vi "FRC myRIO v1.0 Write I2C.vi"(4 "Keep Bus Busy":bool, 6 "Slave Address (7-bit)":u8, 7 "Timeout ms (5)":i32=5, 8 "Error In (No Error)":errorcluster, 9 "Data to Write":u8[](array[numeric])) -> (0 "error out":errorcluster)   [LabVIEW 2017]
uses:
  <vilib>/rvi/errors/niLvFpgaAdjustHostInterfaceError.vi
  <vilib>/Rock Robotics/SystemInterfaces/System/FPGA_SystemFRC FPGA Ref.ctl
  <vilib>/rvi/interface/nirviReadWriteControl/nirviReadWriteControl.xnode
  NiFpgaLv.dll
  <vilib>/rvi/interface/Simulation/niFpgaSimulationCallBeginRW.vi
panel:
  # "This VI writes an array of data to the SPI Data Out register (SPIn.SPDO) and reads an array of data from the SPI Data In register (SPIn.SPDI) for a particular SPI channel (n). The data is written/read one value at a time. Please see Block Diagram for details."
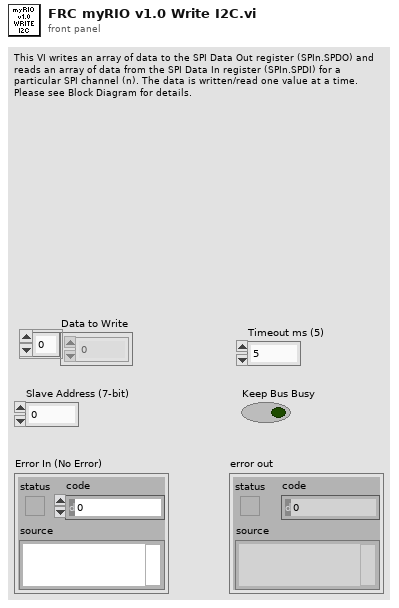
[diagram p1: front panel]
types:
  T1 = typedef "FPGA_SystemFRC FPGA Ref.ctl" = refnum<k20>
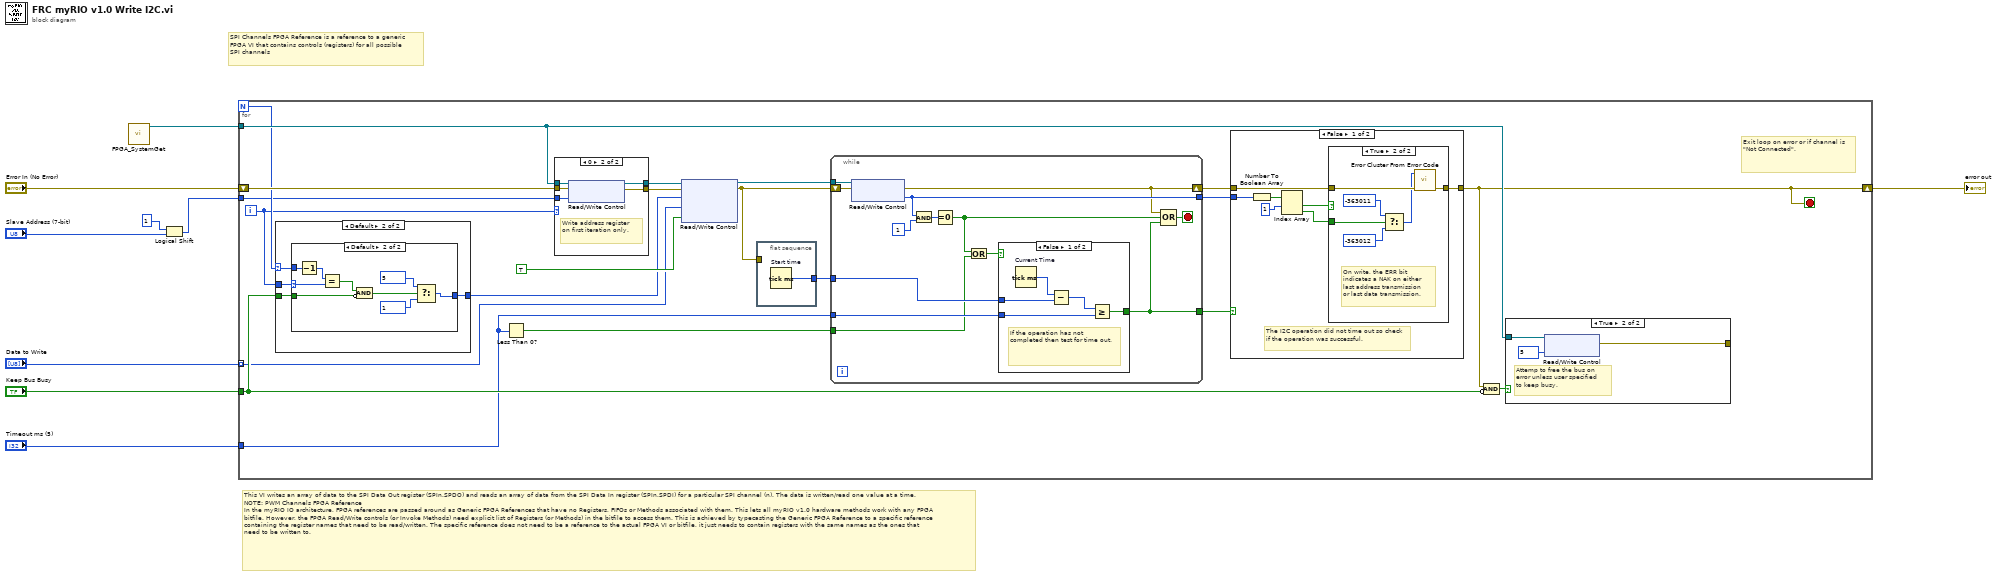
[diagram p0: block diagram]
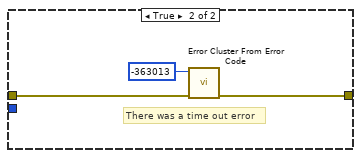
[diagram p3: hidden frame]
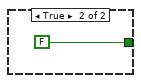
[diagram p6: hidden frame]
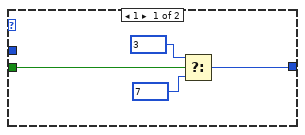
[diagram p7: hidden frame]
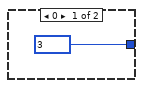
[diagram p8: hidden frame]
diagram:
  # "This VI writes an array of data to the SPI Data Out register (SPIn.SPDO) and reads an array of data from the SPI Data In register (SPIn.SPDI) for a particular SPI channel (n). The data is written/read one value at a time.\nNOTE: PWM Channels FPGA Reference\nIn the myRIO IO architecture, FPGA references are passed around as Generic FPGA References that have no Registers, FIFOs or Methods associated with them. This lets all myRIO v1.0 hardware methods work with any FPGA bitfile. However, the FPGA Read/Write controls (or Invoke Methods) need explicit list of Registers (or Methods) in the bitfile to access them. This is achieved by typecasting the Generic FPGA Reference to a specific reference containing the register names that need to be read/written. The specific reference does not need to be a reference to the actual FPGA VI or bitfile, it just needs to contain registers with the same names as the ones that need to be written to."
  # "SPI Channels FPGA Reference is a reference to a generic FPGA VI that contains controls (registers) for all possible SPI channels"
  n1 = call <vilib>:"FPGA_SystemGet.vi"() -> ("FRC FPGA Ref"=w1:T1)  [unwired: 11 in]
  n2 = Logical Shift(y=i8 1, x="Slave Address (7-bit)") -> (x << y=w4:u8)
  n3 = for {
    N -> [w26]
    shift-right: [w10] -> w6
    shift-left: "Error In (No Error)" -> [w30]
    tunnel: w1 -> [w29]
    tunnel: "Keep Bus Busy" -> [w23]
    tunnel: w4 -> [w25]
    tunnel: "Data to Write" -> [w22] mode=indexing
    tunnel: "Timeout ms (5)" -> [w21]
    i -> [w24]
    stop <- w10 stop-if-true
    # "Exit loop on error or if channel is \"Not Connected\"."
    n4 = case shown="Default" w26 {
      selector: w26 -> [_ w83]
      tunnel: [w81 w84] -> w27
      tunnel: w24 -> [_ w85]
      tunnel: w23 -> [w79 w82]
      frame 1 {
        n5 = Select(t=u8 3 ("y"), s=w79, f=u8 7 ("y")) -> (s? t:f=w81:u8)
      }
      frame Default {
        n6 = case shown="Default" w85 {
          selector: w85 -> [_ w93]
          tunnel: [u8 3 ("y") w87] -> w84
          tunnel: w83 -> [_ w95]
          tunnel: w82 -> [_ w89]
          frame 0 {
          }
          frame Default {
            n7 = Decrement(x=w95) -> (x-1=w94:i32)
            n8 = Equal?(x=w94, y=w93) -> (x = y?=w90:bool)
            n9 = Compound Arithmetic op=AND(w90, invert w89) -> (w88:bool)
            n10 = Select(t=u8 5 ("y"), s=w88, f=u8 1 ("y")) -> (s? t:f=w87:u8)
          }
        }
      }
    }
    n11 = Less Than 0?(x=w21) -> (x < 0?=w20:bool)
    n12 = case shown="0" w24 {
      tunnel: [w53 w58] -> w16
      tunnel: [w52 w57] -> w15
      tunnel: w29 -> [w53 w56]
      tunnel: w30 -> [w52 w55]
      tunnel: w25 -> [_ w54]
      frame Default {
      }
      frame 0 {
        # "Write address register on first iteration only."
        n13 = xnode "Read/Write Control"("FPGA VI Reference In"=w56, "error in"=w55, "Accel.ADDR"=w54) -> ("FPGA VI Reference Out"=w58:T1, "error out"=w57:errorcluster)
      }
    }
    n14 = xnode "Read/Write Control"("FPGA VI Reference In"=w16, "error in"=w15, "Accel.CNTL"=w27, "Accel.DATO"=w22, "Accel.GO"=TRUE ("I2C0.GO")) -> ("FPGA VI Reference Out"=w19:T1, "error out"=w11:errorcluster)
    n15 = flat-sequence {
      tunnel: [w31] -> w13
      tunnel: w11 -> [_]
      frame #0 {
        n16 = Tick Count (ms) "Start time"() -> (millisecond timer value=w31:u32)
      }
    }
    n17 = while {
      tunnel: w19 -> [w70]
      shift-right: [w65] -> w18
      shift-left: w11 -> [w71]
      tunnel: [w66] -> w17
      tunnel: w13 -> [w64]
      tunnel: [w63] -> w12
      tunnel: w21 -> [w62]
      tunnel: w20 -> [w59]
      stop <- w67 stop-if-true
      n18 = xnode "Read/Write Control"("FPGA VI Reference In"=w70, "error in"=w71) -> ("error out"=w65:errorcluster, "Accel.STAT"=w66:u8)  [unwired: 1 out]
      n19 = And(x=w66, y=u8 1) -> (x .and. y?=w68:u8)
      n20 = Equal To 0?(x=w68) -> (x = 0?=w60:bool)
      n21 = Or(x=w60, y=w59) -> (x .or. y?=w61:bool)
      n22 = case shown="False" w61 {
        tunnel: w64 -> [w74 _]
        tunnel: [w73 FALSE] -> w63
        tunnel: w62 -> [w72 _]
        frame False {
          # "If the operation has not completed then test for time out."
          n23 = Tick Count (ms) "Current Time"() -> (millisecond timer value=w75:u32)
          n24 = Subtract(x=w75, y=w74) -> (x-y=w76:u32)
          n25 = Greater Or Equal?(x=w76, y=w72) -> (x >= y?=w73:bool)
        }
        frame True {
        }
      }
      n26 = Compound Arithmetic op=OR(w65, w60, w63) -> (w67:bool)
    }
    n27 = case shown="False" w12 {
      tunnel: w18 -> [w38 w47]
      tunnel: w17 -> [w37 _]
      tunnel: [w33 w46] -> w10
      frame False {
        # "The I2C operation did not time out so check if the operation was successful."
        n28 = Number To Boolean Array(number=w37) -> (Boolean array=w36:bool[])
        n29 = Index Array(array=w36, index #1=1 ("index")) -> (element #1=w35:bool, element #2=w32:bool)  [unwired: 1 in]
        n30 = case shown="True" w35 {
          tunnel: w38 -> [w39 w44]
          tunnel: [w39 w45] -> w33
          tunnel: w32 -> [_ w41]
          frame False {
          }
          frame True {
            # "On write, the ERR bit indicates a NAK on either last address transmission or last data transmission."
            n31 = Select(t=-363011, s=w41, f=-363012) -> (s? t:f=w42:i32)
            n32 = call <vilib>:"Error Cluster From Error Code.vi"("error in (no error)"=w44, "error code (0)"=w42) -> ("error out"=w45:errorcluster)  [unwired: 7 in]
          }
        }
      }
      frame True {
        # "There was a time out error"
        n33 = call <vilib>:"Error Cluster From Error Code.vi"("error in (no error)"=w47, "error code (0)"=-363013) -> ("error out"=w46:errorcluster)  [unwired: 7 in]
      }
    }
    n34 = Compound Arithmetic op=AND(w10, invert w23) -> (w14:bool)
    n35 = case shown="True" w14 {
      tunnel: w29 -> [_ w51]
      tunnel: [_ w49] -> _
      frame False {
      }
      frame True {
        # "Attemp to free the bus on error unless user specified to keep busy."
        n36 = xnode "Read/Write Control"("FPGA VI Reference In"=w51, "Accel.CNTL"=u8 5 ("I2C.C_0.CNTL")) -> ("error out"=w49:errorcluster)  [unwired: 1 in, 1 out]
      }
    }
  }
  "error out" <- w6
